vi "Z6_Beamline_Test.panel.vi"() -> ()   [LabVIEW 2014, in "Z6_Beamline.lvlib"]
doc: "By this VI a hardware switch can be monitored and switched. \n\nThe indicators \"FALSE\", \"TRUE\" and \"SWITCH STATE\" show the value of the Beckhoff-Tag: blue indicates bad tag status reference problems, darkgreen false and lightgreen true. If everything is working fine, \"FALSE\" and \"SWITCH STATE\" should show the same value, while \"TRUE\" has the opposite value. The caption of the sensors for \"FALSE\" and \"TRUE\" are taken out of the database. In case of only one or no sensor these GUI elements are not shown at all.\n\nThe oval button switches. It should be in the same state as the \"SWITCH STATE\" indicator. \n\n\"Delete Instance\" disconnects and removes the instance from the PCS.\n\n\nLicense Agreement for this software:\n\nCopyright (C)\nGesellschaft für Schwerionenforschung, GSI\nPlanckstr. 1\n64291 Darmstadt\nGermany\n\nContact: D.Beck@gsi.de \n\nThis program is free software; you can redistribute it and/or modify it under the terms of the GNU General Public License as published by the Free Software Foundation; either version 2 of the license, or (at your option) any later version.\n\nThis program is distributed in the hope that it will be useful, but WITHOUT ANYW ARRANTY; without even the implied warranty of MERCHANTABILITY or FITNESS FOR A PARTICULAR PURPOSE. See the GNU General License for more details (http://www.gnu.org).\n\nGesellschaft für Schwerionenforschung, GSI\nPlanckstr. 1, 64291 Darmstadt, Germany\nFor all questions and ideas contact: M.Richter@gsi.de, H.Brand@gsi.de or D.Beck@gsi.de.\nLast update: 18-DEC-2002"
uses:
  Z6_Beamline.lvlib
  PH_Basics/PH_Common/Picture/PH_Picture.GUI Element 36x36.ctl
  PH_Basics/PH_Common/Picture/PH_Picture.GUI Element 24x36.ctl
  Z6_Beamline.Switch Instances.ctl
  PH_BL-Master/PH_BL-Master.GUI Refs.ctl
  PH_BL-Master/PH_BL-Master.lvlib
  PH_Basics/PH_Common/PH_Common.lvlib
panel:
  in  "Z6 Switch Instances":T1="N/A"
  in  "Z6_MM10_6PGUI":T2
  in  "Z6_ST_COS_WP_6PWpGUI":T3 caption="Waveplate"
  # "3.40"
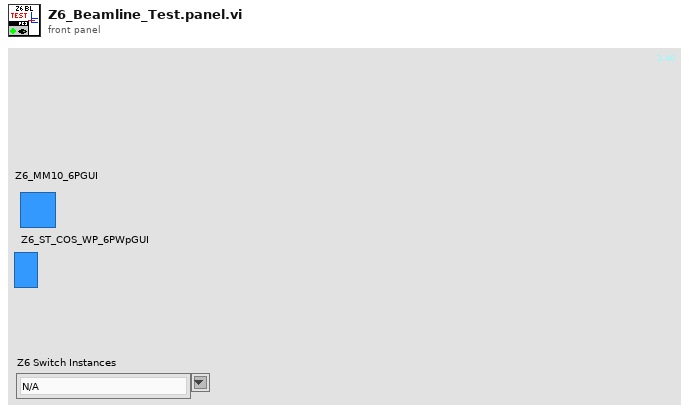
[diagram p1: front panel]
types:
  T1 = typedef "Z6_Beamline.lvlib/Z6_Beamline.Switch Instances.ctl" = string
  T2 = typedef "PH_Common.lvlib/PH_Picture.GUI Element 36x36.ctl" = picture
  T3 = typedef "PH_Common.lvlib/PH_Picture.GUI Element 24x36.ctl" = picture
  T4 = typedef "PH_BL-Master.lvlib/PH_BL-Master.GUI Refs.ctl" = cluster{"Vac GUI Refs":refnum<vi>[], "O2 GUI Refs":refnum<vi>[], "Ready for Shot":refnum<vi>, "Boolean Condition Service Subscriber GUI Refs":refnum<vi>[], "Vision ID on same Node":string, "Picture Condition Service Subscriber GUI Refs":refnum<vi>[], "6P 4Q GUI Refs":refnum<vi>[], "Ref Switch GUI Instances":refnum<vi>, "Ref 6P Switch Instances":refnum<vi>, "Ref BB Instances":refnum<vi>, "Ref Switch Instances":refnum<vi>, "Ref Switch and 6P State Instances":refnum<vi>, "Boolean Status Service Subscriber GUI Refs":refnum<vi>[], "Picture Status Service Subscriber GUI Refs":refnum<vi>[], "Force Sensor Instances":refnum<vi>, "GUI Ref Delete":refnum<vi>}
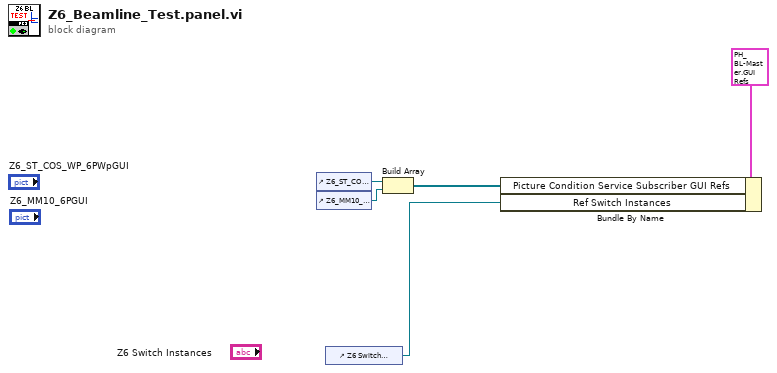
[diagram p0: block diagram]
diagram:
  n1 = control-ref of="Z6_ST_COS_WP_6PWpGUI"() -> (w4:refnum<vi>)
  n2 = control-ref of="Z6_MM10_6PGUI"() -> (w3:refnum<vi>)
  n3 = control-ref of="Z6 Switch Instances"() -> (w1:refnum<vi>)
  n4 = Build Array(w4, w3) -> (w2:refnum<vi>[])
  n5 = Bundle By Name(cluster=T4 {"Vac GUI Refs"=[], "O2 GUI Refs"=[], "Ready for Shot"=refnum, "Boolean Condition Service Subscriber GUI Refs"=[], "Vision ID on same Node"="", "Picture Condition Service Subscriber GUI Refs"=[], "6P 4Q GUI Refs"=[], "Ref Switch GUI Instances"=refnum, "Ref 6P Switch Instances"=refnum, "Ref BB Instances"=refnum, "Ref Switch Instances"=refnum, "Ref Switch and 6P State Instances"=refnum, "Boolean Status Service Subscriber GUI Refs"=[], "Picture Status Service Subscriber GUI Refs"=[], "Force Sensor Instances"=refnum, "GUI Ref Delete"=refnum} ("PH_BL_Master GUI Refs"), "Picture Condition Service Subscriber GUI Refs"=w2, "Ref Switch Instances"=w1) -> ()  [unwired: 1 out]
